vi "GUI.Boolean.GetValue.vi"(8 "error in (no error)":errorcluster, 11 "booleanName":string) -> (0 "error out":errorcluster, 2 "booleanValue":bool)   [LabVIEW 2019]
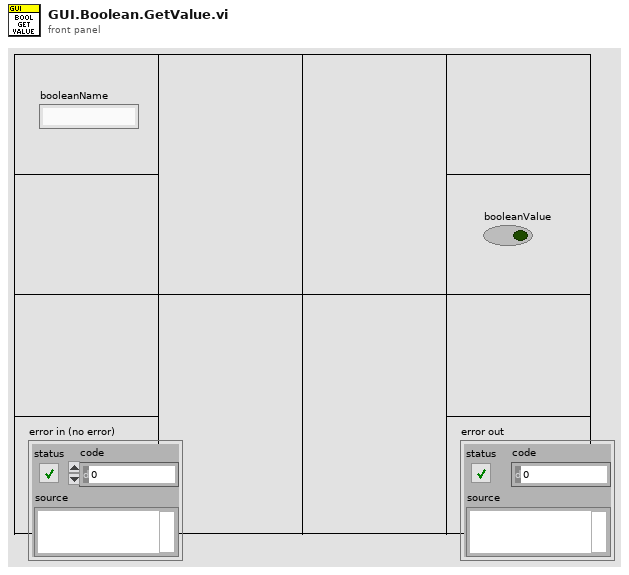
[diagram p1: front panel]
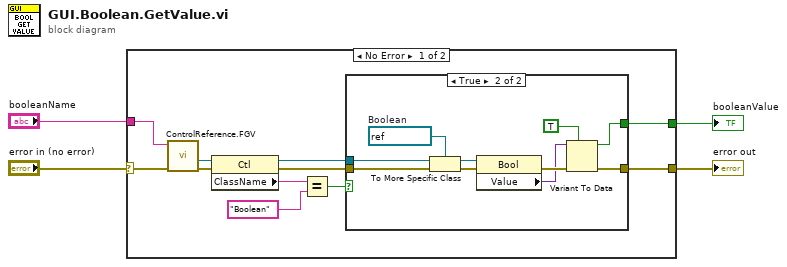
[diagram p0: block diagram]
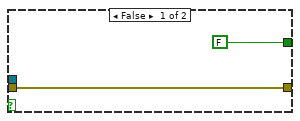
[diagram p2: hidden frame]
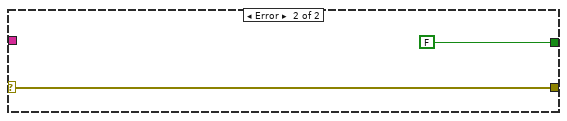
[diagram p3: hidden frame]
diagram:
  n1 = case shown="No Error" "error in (no error)" {
    selector: "error in (no error)" -> [w14 w29]
    tunnel: [w15 w29] -> w2
    tunnel: [w6 FALSE] -> w3
    tunnel: "booleanName" -> [w5 _]
    frame No Error {
      n2 = call "ControlReference.FGV.vi"("error in (no error)"=w14, "controlLabelText"=w5) -> ("error out"=w13:errorcluster, "referenceToControl"=w11:refnum<vi>)  [unwired: 8 in]
      n3 = property class="Ctl"(reference=w11, error in=w13) -> (reference out=w7:refnum<vi>, error out=w12:errorcluster, "ClassName"=w9:string)
      n4 = Equal?(x=w9, y="Boolean") -> (x = y?=w10:bool)
      n5 = case shown="True" w10 {
        tunnel: [w17 w21] -> w15
        tunnel: w12 -> [w17 w24]
        tunnel: w7 -> [_ w23]
        tunnel: [FALSE w18] -> w6
        frame False {
        }
        frame True {
          w27 = refnum<vi> refnum  # Boolean
          n6 = To More Specific Class(target class=w27, reference=w23, error in=w24) -> (specific class reference=w26:refnum<vi>, error out=w25:errorcluster)
          n7 = property class="Bool"(reference=w26, error in=w25) -> (error out=w22:errorcluster, "Value"=w19:variant)  [unwired: 1 out]
          n8 = Variant To Data(error in=w22, type=TRUE, Variant=w19) -> (data=w18:bool, error out=w21:errorcluster)
        }
      }
    }
    frame Error {
    }
  }
  "booleanValue" <- w3
  "error out" <- w2
